vi "力特性 推力对应扭矩.vi"(7 "推力":dbl=136.0 format="%#_13g", 8 "扭矩左":dbl[](array[numeric]), 9 "扭矩右":dbl[](array[numeric]), 10 "推力左":dbl[](array[numeric]), 11 "推力右":dbl[](array[numeric])) -> (2 "推力左扭矩":dbl, 3 "推力右扭矩":dbl)   [LabVIEW 2015, in "Logging.lvlib"]
uses:
  Logging.lvlib
panel:
  out "波形图 2":dbl[](graph)
  out "波形图":dbl[](graph)
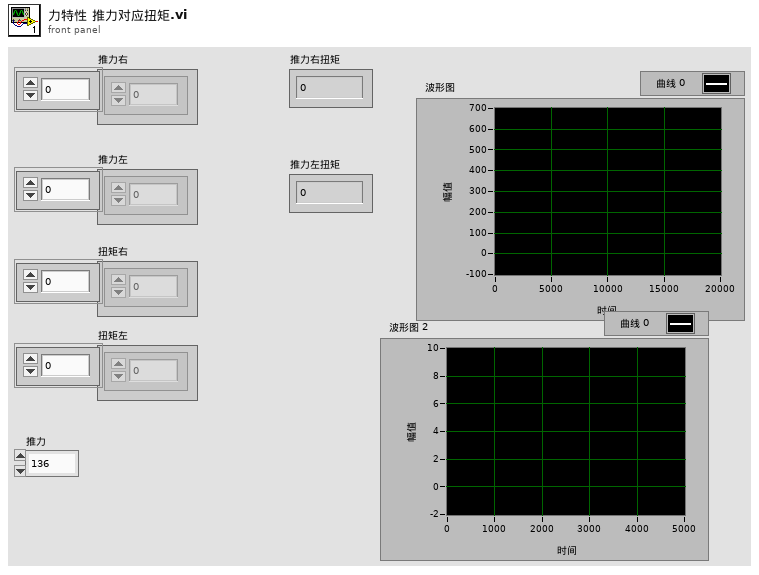
[diagram p1: front panel]
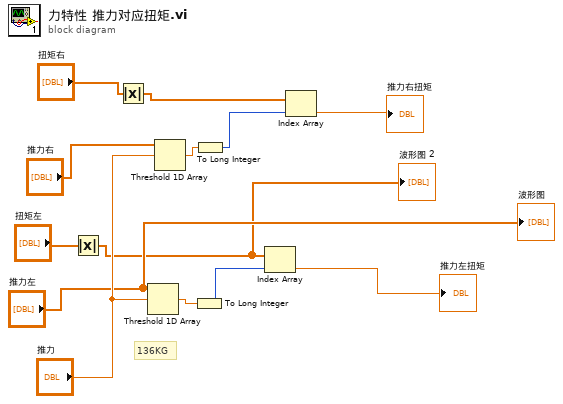
[diagram p0: block diagram]
diagram:
  # "136KG"
  n1 = Absolute Value(x="扭矩左") -> (abs(x)=w1:dbl[])
  "波形图 2" <- w1
  n2 = Absolute Value(x="扭矩右") -> (abs(x)=w3:dbl[])
  n3 = Threshold 1D Array(2:"推力", 3:"推力左") -> (0:w13:dbl)  [unwired: 1 in]
  n4 = Threshold 1D Array(2:"推力", 3:"推力右") -> (0:w9:dbl)  [unwired: 1 in]
  n5 = To Long Integer(number=w13) -> (32bit integer=w12:i32)
  n6 = To Long Integer(number=w9) -> (32bit integer=w7:i32)
  n7 = Index Array(array=w1, index=w12) -> (element=→"推力左扭矩":dbl)
  n8 = Index Array(array=w3, index=w7) -> (element=→"推力右扭矩":dbl)
  "波形图" <- "推力左"
